vi "Connect Database.vi"(8 "error in (no error)":errorcluster) -> (0 "error out":errorcluster, 3 "connection reference":T1)   [LabVIEW 2015, in "Database Processing.lvlib"]
uses:
  Database Processing.lvlib
  <vilib>/addons/database/Connection.llb/Conn ObjectReference.ctl
  <vilib>/addons/database/Connection.llb/DB Tools Open Connec (String).vi
  <vilib>/addons/database/NI_Database_API.lvlib
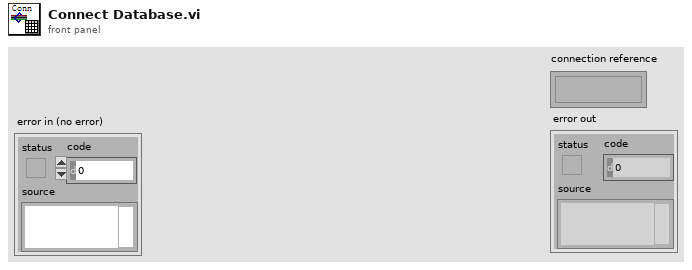
[diagram p1: front panel]
types:
  T1 = typedef "NI_Database_API.lvlib/Conn ObjectReference.ctl" = refnum<k1>
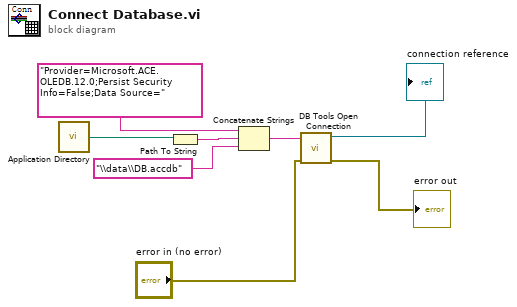
[diagram p0: block diagram]
diagram:
  n1 = call <vilib>:"Application Directory.vi"() -> ("Application Directory"=w7:path)
  n2 = Path To String(path=w7) -> (string=w4:string)
  n3 = Concatenate Strings("Provider=Microsoft.ACE.OLEDB.12.0;Persist Security Info=False;Data Source=" ("字符串"), w4, "\\data\\DB.accdb" ("字符串")) -> (w5:string)
  n4 = call-poly <vilib>:"DB Tools Open Connection.vi"("error in (no error)"="error in (no error)", "connection information"=w5) -> ("error out"=→"error out":errorcluster, "connection reference"=→"connection reference":T1)  [unwired: 6 in]
